vi "Script_Create Steering Wheel.vi"(6 "error source terminal refnum":refnum<vi>, 8 "error in (no error)":errorcluster, 10 "owner diagram refnum":refnum<vi>, 11 "wheel in":refnum<class "NI_Robotics_Wheel.lvclass">) -> (0 "error out":errorcluster, 1 "created?":bool, 2 "wheel out terminal refnum":refnum<vi>, 4 "error out terminal refnum":refnum<vi>)   [LabVIEW 2017, in "NI_Robotics_Scripting Utilities.lvlib"]
uses:
  <vilib>/robotics/Utilities/Scripting/NI_Robotics_Scripting Utilities.lvlib
  <vilib>/robotics/Steering/Wheel/NI_Robotics_Wheel.lvclass
  <vilib>/Utility/miscctls.llb/LVPointTypeDef.ctl
  <vilib>/robotics/Steering/Steering Wheel/Create Steering Wheel.vi
  <vilib>/robotics/Steering/Steering Wheel/NI_Robotics_Steering Wheel.lvclass
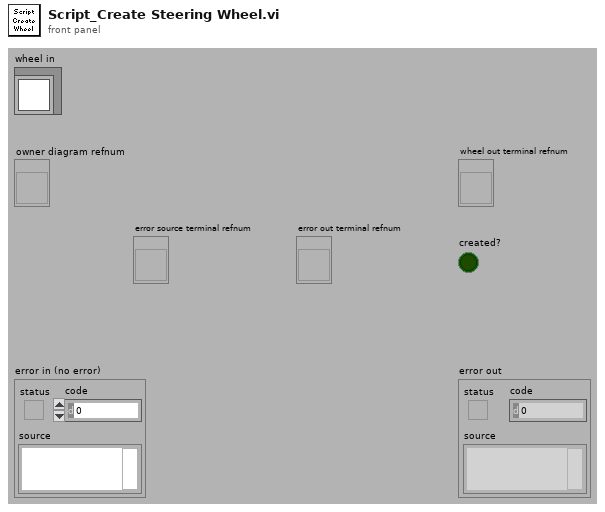
[diagram p1: front panel]
types:
  T1 = typedef "LVPointTypeDef.ctl" = cluster{"Horizontal":i16, "Vertical":i16}
  T2 = typedef "NI_Robotics_Wheel.lvclass/Wheel Parameters.ctl" = cluster{"wheel radius":dbl, "gear ratio":dbl, "forward rotation direction":T3}
  T3 = typedef "NI_Robotics_Wheel.lvclass/Rotation Direction.ctl" = u16
  T4 = typedef "NI_Robotics_Steering Wheel.lvclass/Steering Wheel Parameters.ctl" = cluster{"steering gear ratio":dbl, "motor angle offset (rad)":dbl, "steering angle range":T5}
  T5 = typedef "NI_Robotics_Steering Wheel.lvclass/Steering Angle Range.ctl" = cluster{"min steering angle (rad)":dbl, "max steering angle (rad)":dbl}
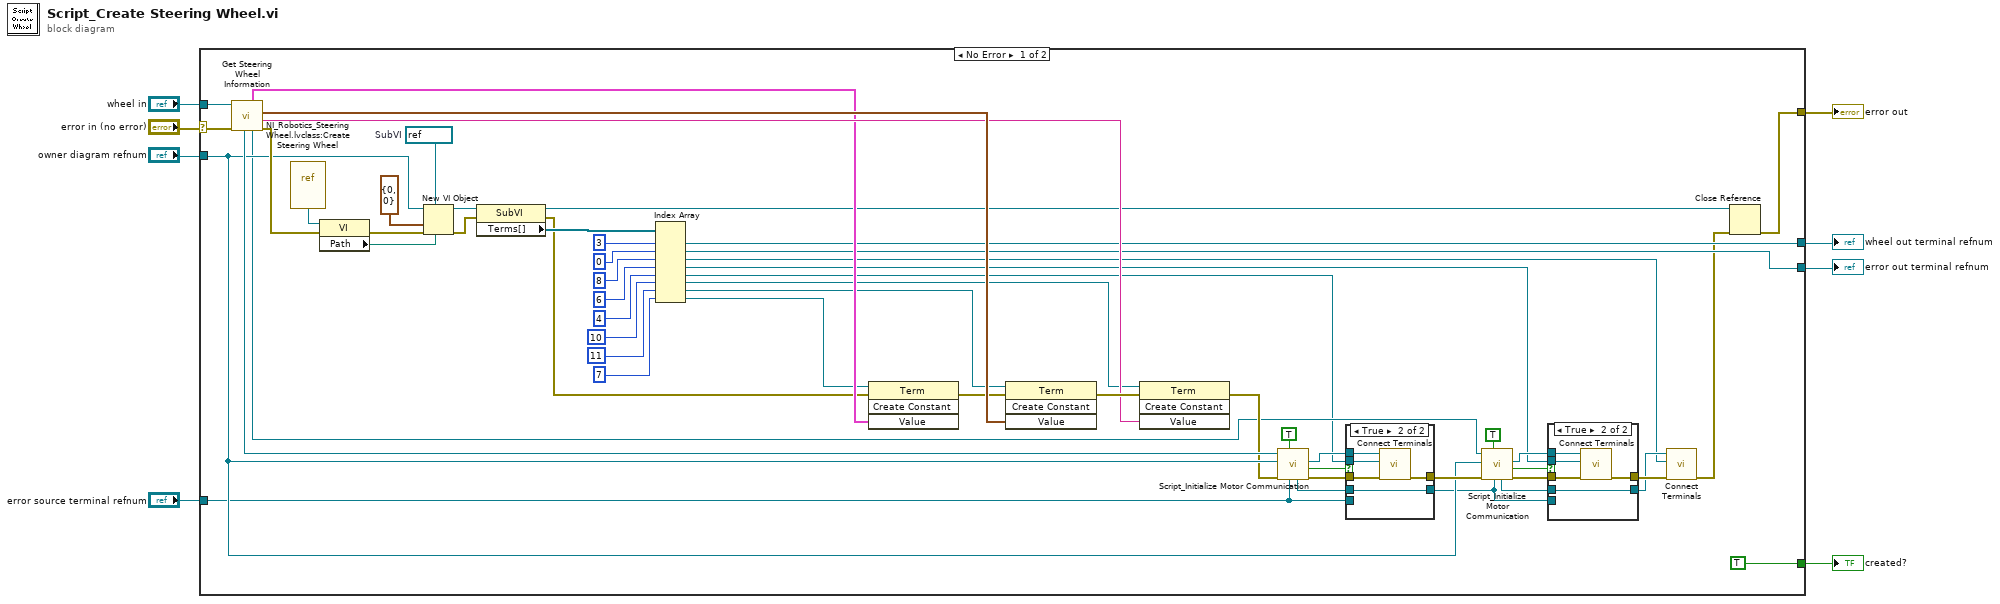
[diagram p0: block diagram]
diagram:
  n1 = case shown="No Error" "error in (no error)" {
    selector: "error in (no error)" -> [w63 w79]
    tunnel: "wheel in" -> [w64 _]
    tunnel: [w9 w79] -> w5
    tunnel: "owner diagram refnum" -> [w46 _]
    tunnel: [w14 _] -> w3
    tunnel: [w12 _] -> w2
    tunnel: [TRUE _] -> w4
    tunnel: "error source terminal refnum" -> [w40 _]
    frame No Error {
      w62 = refnum<vi> refnum  # SubVI
      n2 = call <vilib>:"Get Steering Wheel Information.vi"("error in (no error)"=w63, "wheel in"=w64) -> ("error out"=w54:errorcluster, "wheel name"=w55:string, "wheel parameters"=w56:T2, "motor communication"=w39:refnum<class "NI_Robotics_Motor Communication.lvclass">, "steering parameters"=w51:T4, "steering motor communication"=w48:refnum<class "NI_Robotics_Motor Communication.lvclass">)  [unwired: 3 in, 1 out]
      n3 = vi-ref "NI_Robotics_Steering Wheel.lvclass:Create Steering Wheel.vi"() -> (w57:refnum<vi>)
      n4 = property class="VI"(reference=w57, error in=w54) -> (error out=w61:errorcluster, "Path"=w58:path)  [unwired: 1 out]
      n5 = New VI Object(vi object class=w62, owner refnum=w46, position/next to=T1 {"Horizontal"=0, "Vertical"=0} ("relative position/next to refnum"), 6:w58, 8:w61) -> (object refnum=w31:refnum<vi>, 0:w29:errorcluster)  [unwired: 3 in]
      n6 = property class="SubVI"(reference=w31, error in=w29) -> (reference out=w11:refnum<vi>, error out=w28:errorcluster, "Terms[]"=w30:refnum<vi>[])
      n7 = Index Array(array=w30, index #1=3 ("index"), index #2=0 ("index"), index #3=8 ("index"), index #4=6 ("index"), index #5=4 ("index"), index #6=10 ("index"), index #7=11 ("index"), index #8=7 ("index")) -> (element #1=w12:refnum<vi>, element #2=w14:refnum<vi>, element #3=w16:refnum<vi>, element #4=w18:refnum<vi>, element #5=w19:refnum<vi>, element #6=w22:refnum<vi>, element #7=w24:refnum<vi>, element #8=w26:refnum<vi>)
      n8 = invoke class="Term" method="Create Constant"(reference=w26, error in=w28, "Value"=w51) -> (error out=w52:errorcluster)  [unwired: 1 in, 3 out]
      n9 = invoke class="Term" method="Create Constant"(reference=w24, error in=w52, "Value"=w56) -> (error out=w59:errorcluster)  [unwired: 1 in, 3 out]
      n10 = invoke class="Term" method="Create Constant"(reference=w22, error in=w59, "Value"=w55) -> (error out=w43:errorcluster)  [unwired: 1 in, 3 out]
      n11 = call <vilib>:"Script_Initialize Motor Communication.vi"("error source terminal refnum"=w40, "skip if name is empty (F)"=TRUE, "error in (no error)"=w43, "owner diagram refnum"=w46, "motor communication in"=w48) -> ("error out"=w42:errorcluster, "created?"=w45:bool, "motor communication out terminal refnum"=w44:refnum<vi>, "error out terminal refnum"=w41:refnum<vi>)  [unwired: 2 in, 1 out]
      n12 = case shown="True" w45 {
        tunnel: w44 -> [_ w77]
        tunnel: w42 -> [w73 w78]
        tunnel: w40 -> [w72 _]
        tunnel: [w73 w76] -> w49
        tunnel: w41 -> [_ w75]
        tunnel: [w72 w75] -> w34
        tunnel: w19 -> [_ w74]
        frame False {
        }
        frame True {
          n13 = call <vilib>:"Connect Terminals.vi"("error in (no error)"=w78, "sink terminal"=w74, "source terminal"=w77) -> ("error out"=w76:errorcluster)  [unwired: 7 in, 1 out]
        }
      }
      n14 = call <vilib>:"Script_Initialize Motor Communication.vi"("error source terminal refnum"=w34, "skip if name is empty (F)"=TRUE, "error in (no error)"=w49, "owner diagram refnum"=w46, "motor communication in"=w39) -> ("error out"=w36:errorcluster, "created?"=w38:bool, "motor communication out terminal refnum"=w37:refnum<vi>, "error out terminal refnum"=w35:refnum<vi>)  [unwired: 2 in, 1 out]
      n15 = case shown="True" w38 {
        tunnel: w37 -> [_ w70]
        tunnel: w36 -> [w66 w71]
        tunnel: w34 -> [w65 _]
        tunnel: [w66 w69] -> w33
        tunnel: w35 -> [_ w68]
        tunnel: [w65 w68] -> w32
        tunnel: w18 -> [_ w67]
        frame False {
        }
        frame True {
          n16 = call <vilib>:"Connect Terminals.vi"("error in (no error)"=w71, "sink terminal"=w67, "source terminal"=w70) -> ("error out"=w69:errorcluster)  [unwired: 7 in, 1 out]
        }
      }
      n17 = call <vilib>:"Connect Terminals.vi"("error in (no error)"=w33, "sink terminal"=w16, "source terminal"=w32) -> ("error out"=w10:errorcluster)  [unwired: 7 in, 1 out]
      n18 = Close Reference(reference=w11, error in (no error)=w10) -> (error out=w9:errorcluster)
    }
    frame Error {
    }
  }
  "error out" <- w5
  "wheel out terminal refnum" <- w2
  "error out terminal refnum" <- w3
  "created?" <- w4
